vi "Unsubscribe.vi"(8 "error in (no error)":errorcluster, 9 "Unique Subscriber ID":string, 10 "Subscription Name":string, 11 "Mediator In":refnum<class "IMediator.lvclass">) -> (0 "error out":errorcluster, 3 "Mediator Out":refnum<class "IMediator.lvclass">)   [LabVIEW 2015, in "IMediator.lvlib" / "IMediator.lvclass"]
uses:
  IMediator.lvclass
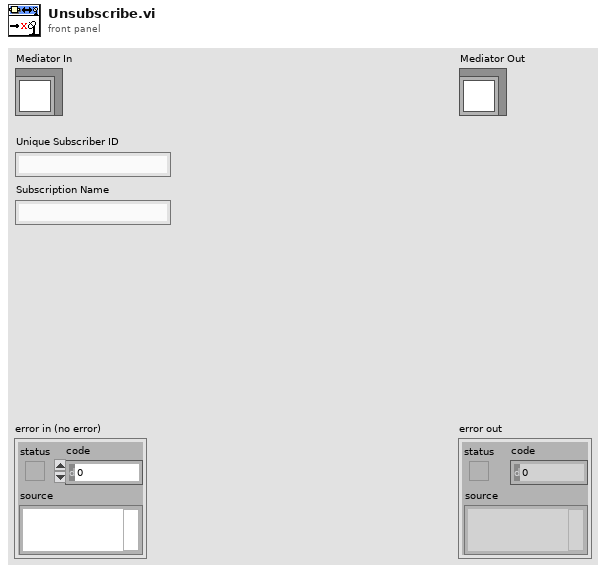
[diagram p1: front panel]
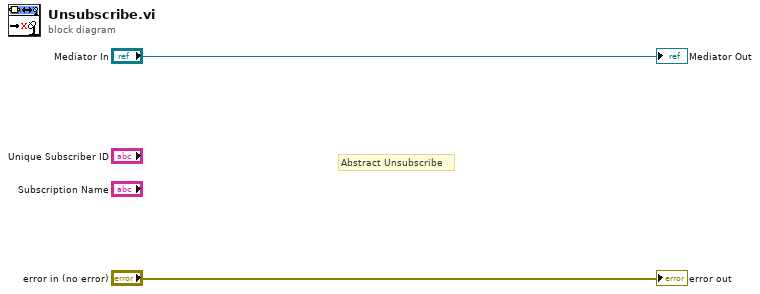
[diagram p0: block diagram]
diagram:
  # "Abstract Unsubscribe"
  "error out" <- "error in (no error)"
  "Mediator Out" <- "Mediator In"
